vi "LED_I2C_setPWM.vi"(0 "Servo Controller Index":u8, 5 "PWM Channel":u8, 7 "On (0)":u16, 9 "Off (duty-cycle)":u16, 11 "Error In":errorcluster) -> (15 "Error Out":errorcluster)   [LabVIEW 2013]
uses:
  <vilib>/myRIO/Instrument Drivers/Onboard IO/I2C/vis/Smart Open.vi
  <vilib>/myRIO/Instrument Drivers/Onboard IO/I2C/vis/Configure.vi
  <vilib>/myRIO/Instrument Drivers/Onboard IO/I2C/vis/Write.vi
  <vilib>/myRIO/Instrument Drivers/Onboard IO/I2C/vis/Open.vi
  <vilib>/myRIO/Common/Instrument Driver Framework/myRIO v1.0/I2C/vis/myRIO v1.1 Open I2C.vi
  <vilib>/myRIO/Common/Instrument Driver Framework/Utilities/vis/Validate Channels.vi
  <vilib>/myRIO/Common/Instrument Driver Framework/myRIO v1.0/I2C/vis/myRIO v1.0 Reserve I2C.vi
  <vilib>/myRIO/Common/Instrument Driver Framework/myRIO v1.0/I2C/vis/myRIO v1.0 Build MUX Configuration I2C.vi
  <vilib>/myRIO/Common/Instrument Driver Framework/myRIO v1.0/Resource Manager/vis/myRIO v1.0 Reserve Channel List.vi
  <vilib>/myRIO/Common/Instrument Driver Framework/myRIO v1.0/Resource Manager/vis/myRIO v1.0 Create Configuration List.vi
  <vilib>/myRIO/Common/Instrument Driver Framework/myRIO v1.0/Resource Manager/vis/myRIO v1.0 Reserve Channel.vi
  <vilib>/myRIO/Common/Instrument Driver Framework/myRIO v1.0/Resource Manager/vis/myRIO v1.0 Unreserve Channel.vi
  <vilib>/myRIO/Common/Instrument Driver Framework/myRIO v1.0/Resource Manager/vis/myRIO v1.0 Build Mutex Name.vi
  <vilib>/myRIO/Common/Instrument Driver Framework/myRIO v1.0/myRIO v1.1 Open.vi
  <vilib>/Utility/VariantDataType/GetNumericInfo.vi
  <vilib>/Utility/error.llb/Error Cluster From Error Code.vi
  <vilib>/myRIO/Common/Instrument Driver Framework/Utilities/vis/IO Manager.vi
  <vilib>/myRIO/Common/Instrument Driver Framework/Utilities/vis/Configuration Manager.vi
  <vilib>/myRIO/Common/Instrument Driver Framework/myRIO v1.0/Resource Manager/vis/myRIO v1.0 Configure IO.vi
  <vilib>/myRIO/Common/Instrument Driver Framework/myRIO v1.0/myRIO v1.0 Close.vi
  <vilib>/myRIO/Common/Instrument Driver Framework/myRIO v1.0/I2C/vis/myRIO v1.0 Configure I2C.vi
  <vilib>/myRIO/Common/Instrument Driver Framework/myRIO v1.0/I2C/vis/myRIO v1.0 Write I2C.vi
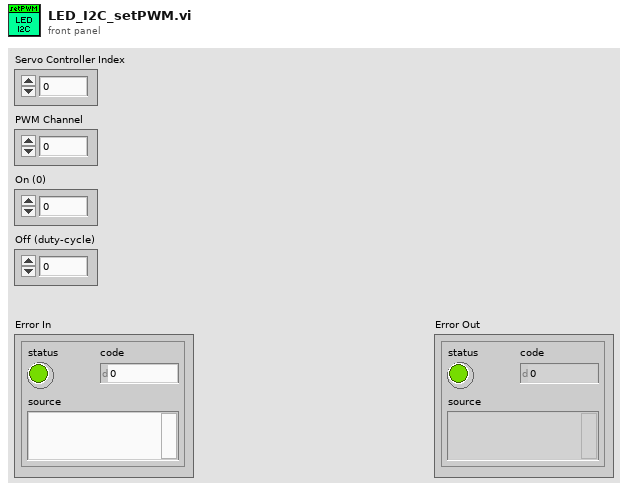
[diagram p1: front panel]
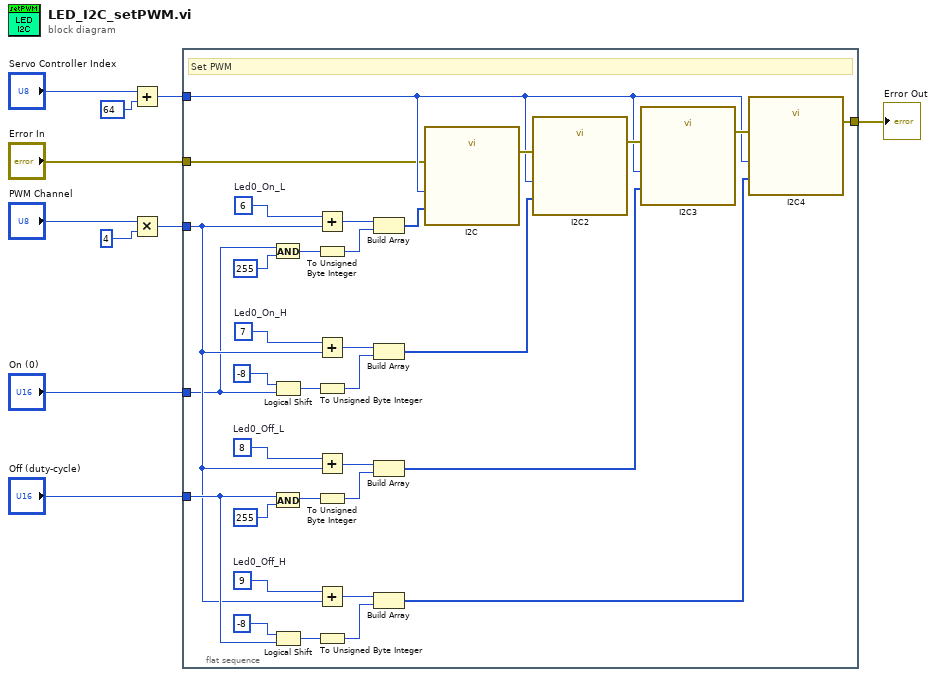
[diagram p0: block diagram]
diagram:
  n1 = Add(x="Servo Controller Index", y=u8 64 ("Slave Address (7-bit)")) -> (x+y=w9:u8)
  n2 = Multiply(x="PWM Channel", y=u8 4) -> (x*y=w7:u8)
  n3 = flat-sequence {
    tunnel: w9 -> [w14]
    tunnel: [w24] -> w2
    tunnel: w7 -> [w13]
    tunnel: "On (0)" -> [w12]
    tunnel: "Off (duty-cycle)" -> [w28]
    tunnel: "Error In" -> [w11]
    frame #0 {
      w40 = u8 9  # Led0_Off_H
      w41 = u8 8  # Led0_Off_L
      w42 = u8 7  # Led0_On_H
      w43 = u8 6  # Led0_On_L
      # "Set PWM"
      n4 = And(x=w12, y=u16 255) -> (x .and. y?=w36:u16)
      n5 = Logical Shift(y=i8 -8 ("x"), x=w12) -> (x << y=w35:u16)
      n6 = And(x=w28, y=u16 255) -> (x .and. y?=w33:u16)
      n7 = Logical Shift(y=i8 -8 ("x"), x=w28) -> (x << y=w30:u16)
      n8 = Add(x=w43, y=w13) -> (x+y=w39:u8)
      n9 = To Unsigned Byte Integer(number=w36) -> (unsigned 8bit integer=w37:u8)
      n10 = Add(x=w42, y=w13) -> (x+y=w23:u8)
      n11 = To Unsigned Byte Integer(number=w35) -> (unsigned 8bit integer=w22:u8)
      n12 = Add(x=w41, y=w13) -> (x+y=w19:u8)
      n13 = To Unsigned Byte Integer(number=w33) -> (unsigned 8bit integer=w18:u8)
      n14 = Add(x=w40, y=w13) -> (x+y=w17:u8)
      n15 = To Unsigned Byte Integer(number=w30) -> (unsigned 8bit integer=w16:u8)
      n16 = Build Array(w39, w37) -> (w29:u8[])
      n17 = Build Array(w23, w22) -> (w21:u8[])
      n18 = Build Array(w19, w18) -> (w20:u8[])
      n19 = Build Array(w17, w16) -> (w15:u8[])
      n20 = call "I2C"("Slave Address (7-bit)"=w14, "Bytes to Write"=w29, "error in (no error)"=w11) -> ("error out"=w27:errorcluster)  [unwired: 24 in]
      n21 = call "I2C2"("Slave Address (7-bit)"=w14, "Bytes to Write"=w21, "error in (no error)"=w27) -> ("error out"=w26:errorcluster)  [unwired: 24 in]
      n22 = call "I2C3"("Slave Address (7-bit)"=w14, "Bytes to Write"=w20, "error in (no error)"=w26) -> ("error out"=w25:errorcluster)  [unwired: 24 in]
      n23 = call "I2C4"("Slave Address (7-bit)"=w14, "Bytes to Write"=w15, "error in (no error)"=w25) -> ("error out"=w24:errorcluster)  [unwired: 24 in]
    }
  }
  "Error Out" <- w2
